vi "velocidad.vi"() -> ()   [LabVIEW 2013]
panel:
  out "distancia":dbl
  out "tiempo":i16
  in  "posicion inicial":dbl
  in  "velocidad":dbl
  in  "stop":bool
  in  "aceleracion":dbl
  in  "Boolean":bool
  out "Waveform Chart":cluster{"y":dbl, "y2":dbl}(graph)
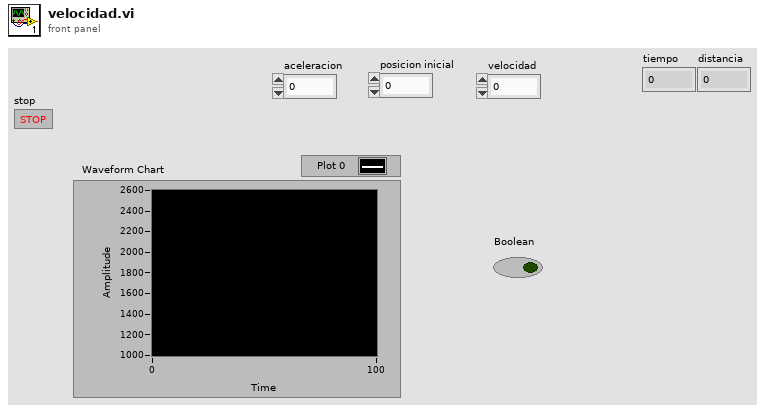
[diagram p1: front panel]
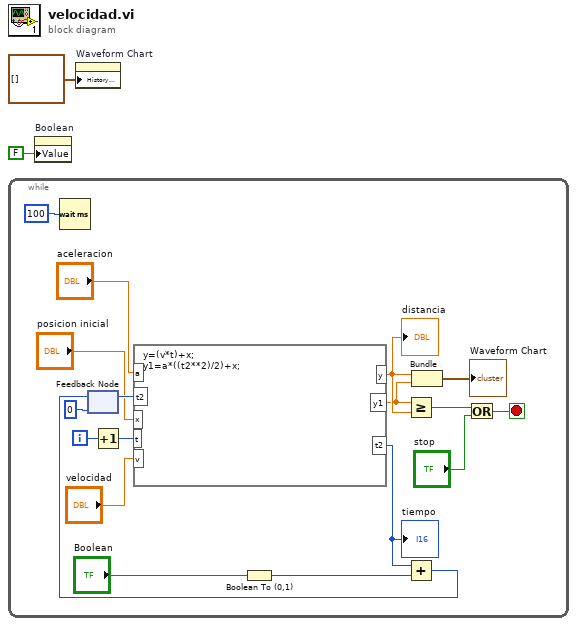
[diagram p0: block diagram]
diagram:
  n1 = while {
    i -> [w19]
    stop <- w8 stop-if-true
    n2 = Wait (ms)(milliseconds to wait=u32 100) -> ()  [unwired: 1 out]
    n3 = feedback #1(i16 0) -> (w13:i16)
    n4 = Increment(x=w19) -> (x+1=w18:i32)
    n5 = formula code="y=(v*t)+x;\ny1=a*((t2**2)/2)+x;"("t"=w18, "t2"=w13, "a"="aceleracion", "v"="velocidad", "x"="posicion inicial") -> ("t2"=w15:i16, "y1"=w6:dbl, "y"=w7:dbl)
    "tiempo" <- w15
    "distancia" <- w7
    n6 = Boolean To (0,1)(Boolean="Boolean") -> (0, 1=w16:i16)
    n7 = Greater Or Equal?(x=w6, y=w7) -> (x >= y?=w9:bool)
    n8 = Add(x=w15, y=w16) -> (x+y=w14:i16)
    n9 = feedback-in #1(w14) -> ()
    n10 = Bundle("y"=w7, "y1"=w6) -> (→"Waveform Chart":cluster{"y":dbl, "y1":dbl})  [unwired: 1 in]
    n11 = Or(x=w9, y="stop") -> (x .or. y?=w8:bool)
  }
  n12 = property on="Boolean" class="Bool (strict)"("Value"=FALSE ("Boolean")) -> ()  [unwired: 2 in, 2 out]
  n13 = property on="Waveform Chart" class="WFChart (strict)"("History Data"=cluster{"y":dbl, "y2":dbl}[] []) -> ()  [unwired: 2 in, 2 out]
